vi "Drive Globals.vi"() -> ()   [LabVIEW 2016]
uses:
  Drive Notifier.ctl
  Drive Control Type.ctl
panel:
  in  "Right Back Initial Position":dbl
  in  "Right Front Initial Position":dbl
  in  "Left Back Initial Position":dbl
  in  "Left Front Initial Position":dbl
  in  "Pigeon IMU":string="Pigeon IMU"
  in  "Right Back Wheel Spin":string="Right Back Wheel Spin"
  in  "Right Front Wheel Spin":string="Right Front Wheel Spin"
  in  "Left Front Wheel Spin":string="Left Front Wheel Spin"
  in  "Left Back Wheel Spin":string="Left Back Wheel Spin"
  in  "Right Back Wheel Drive":string="Right Back Wheel Drive"
  in  "Right Front Wheel Drive":string="Right Front Wheel Drive"
  in  "Left Front Wheel Drive":string="Left Front Wheel Drive"
  in  "Left Back Wheel Drive":string="Left Back Wheel Drive"
  in  "Robot Heading":dbl
  in  "Left Back Wheel Amplification Factor":dbl=1.0
  in  "Left Front Wheel Amplification Factor":dbl=1.0
  in  "Front Left Wheel Angle":dbl
  in  "Front Right Wheel Angle":dbl
  in  "Back Left Wheel Angle":dbl
  in  "Back Right Wheel Angle":dbl
  in  "Bang-Bang Swerve Twist Motor Power":dbl
  in  "Bang-Bang Swerve Angle Deadband":dbl
  in  "Drive DVR":refnum<data-value>
  in  "Drive Notifier":refnum<notifier>
  # "These refnums are for the writing and creation\nof the drive subsystem's data."
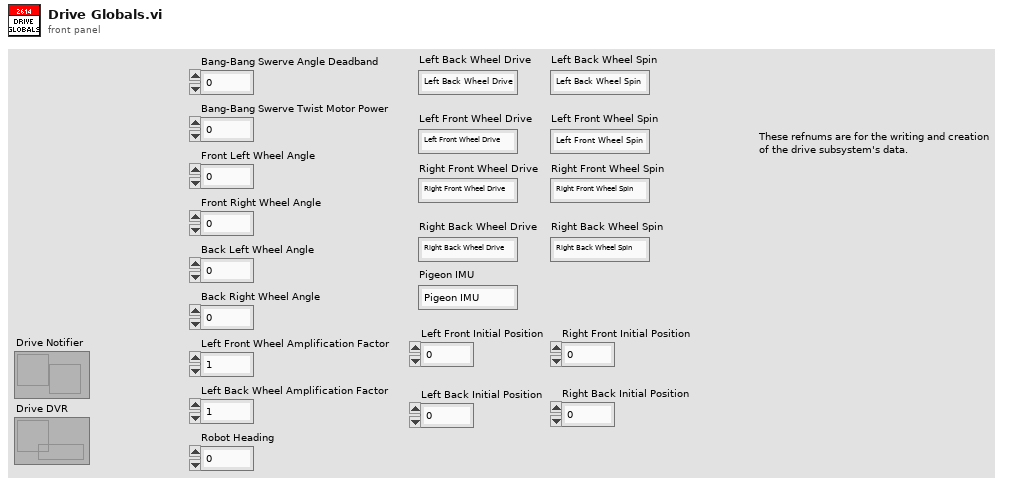
[diagram p1: front panel]
diagram:
